vi "TestBooleenColor.vi"() -> ()   [LabVIEW 2020]
panel:
  in  "Colors [4] 3":cluster{u32, u32}[](array[cluster])=[{9868950, 9868950}, {13816530, 13816530}, {9868950, 9868950}, {13816530, 13816530}]
  in  "Checkbox":bool
  in  "Button":bool
  in  "Boolean 3":bool
  in  "Colors [4] 2":cluster{u32, u32}[](array[cluster])
  in  "Boolean 2":bool
  in  "Colors [4]":cluster{u32, u32}[](array[cluster])
  in  "Boolean":bool
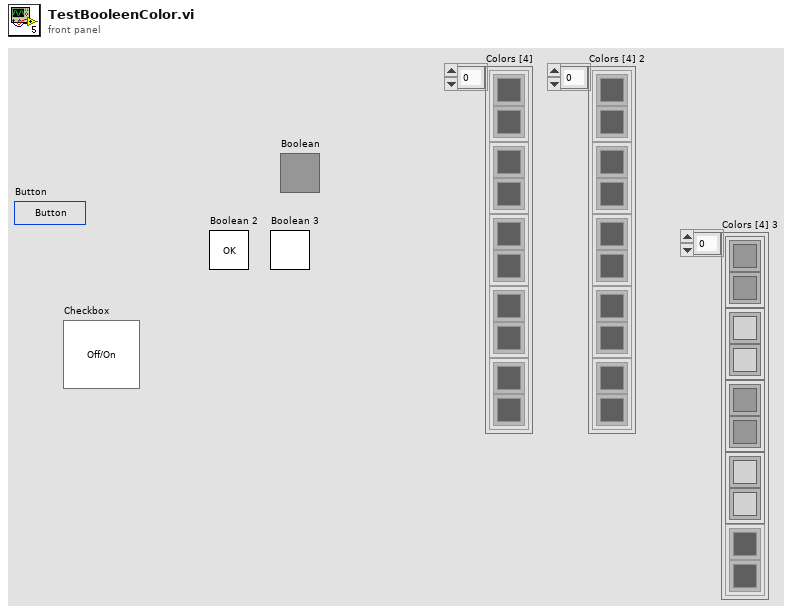
[diagram p1: front panel]
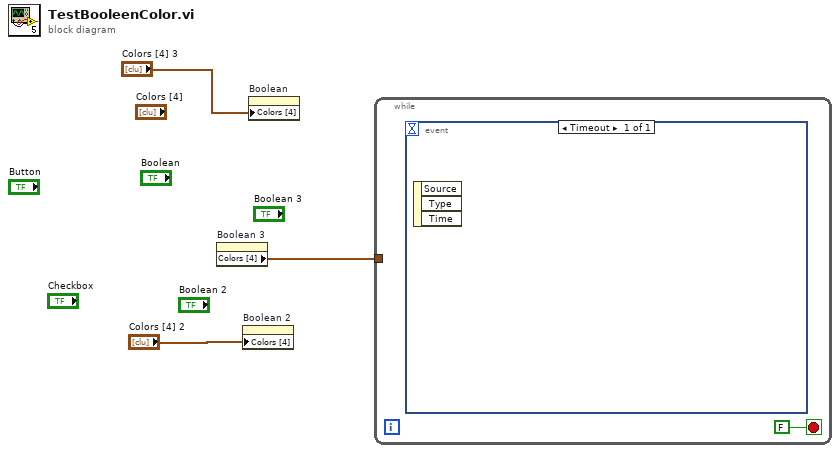
[diagram p0: block diagram]
diagram:
  n1 = property on="Boolean 3" class="Bool"() -> ("Colors [4]"=w2:cluster{u32, u32}[])  [unwired: 2 in, 2 out]
  n2 = property on="Boolean 2" class="Bool"("Colors [4]"="Colors [4] 2") -> ()  [unwired: 2 in, 2 out]
  n3 = property on="Boolean" class="Bool (strict)"("Colors [4]"="Colors [4] 3") -> ()  [unwired: 2 in, 2 out]
  n4 = while {
    tunnel: w2 -> [_]
    stop <- FALSE stop-if-true
    n5 = event shown="[0] Timeout" {
      selector: _ -> [_]
      dyn-events: _ -> [_]
      timeout: _ -> [_]
      event Timeout {
        n6 = event-data() -> ()  [unwired: 1 in, 3 out]
      }
    }
  }
